vi "PQ_flags.vi"() -> ()   [LabVIEW 2018]
panel:
  in  "g6_trans_flag":bool
  in  "g6_swell_flag":bool
  in  "g6_sag_flag":bool
  in  "g5_trans_flag":bool
  in  "g5_swell_flag":bool
  in  "g5_sag_flag":bool
  in  "g4_trans_flag":bool
  in  "g4_swell_flag":bool
  in  "g4_sag_flag":bool
  in  "g3_trans_flag":bool
  in  "g3_swell_flag":bool
  in  "g3_sag_flag":bool
  in  "g2_trans_flag":bool
  in  "g2_swell_flag":bool
  in  "g2_sag_flag":bool
  in  "g1_trans_flag":bool
  in  "g1_swell_flag":bool
  in  "g1_sag_flag":bool
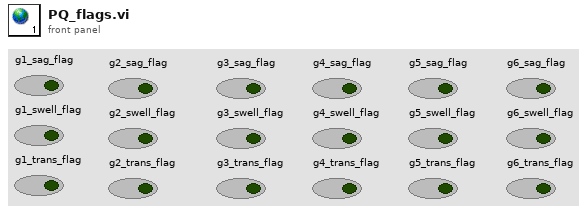
[diagram p1: front panel]
diagram:
